vi "test2.vi"(1 "Numeric 3":i32, 2 "Numeric in":i32) -> (0 "Numeric out":i32)   [LabVIEW 2016]
doc: "(x+y)*x-x"
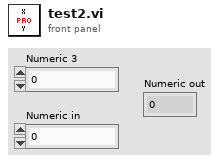
[diagram p1: front panel]
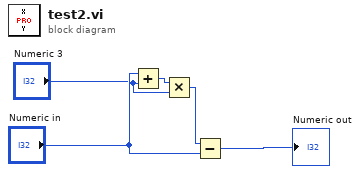
[diagram p0: block diagram]
diagram:
  n1 = Add(x="Numeric in", y="Numeric 3") -> (x+y=w1:i32)
  n2 = Multiply(x=w1, y="Numeric 3") -> (x*y=w3:i32)
  n3 = Subtract(x=w3, y="Numeric in") -> (x-y=→"Numeric out":i32)
